vi "Read Environment Options.vi"(8 "error in (no error)":errorcluster, 11 "WebView2 Control in":refnum<class "WebView2 QControl.lvclass">) -> (0 "error out":errorcluster, 2 "Env Options":T1, 3 "WebView2 Control out":refnum<class "WebView2 QControl.lvclass">)   [LabVIEW 2020, in "WebView2 QControl.lvlib" / "WebView2 QControl.lvclass"]
uses:
  WebView2 QControl.lvclass
  WebView2 QControl.lvclass/WebView2 QControl.ctl
  Webview2 Lib/WebView2 Control Object/WebView2 Control.lvclass
  Webview2 Lib/WebView2 Control Object/Core Env Options.ctl
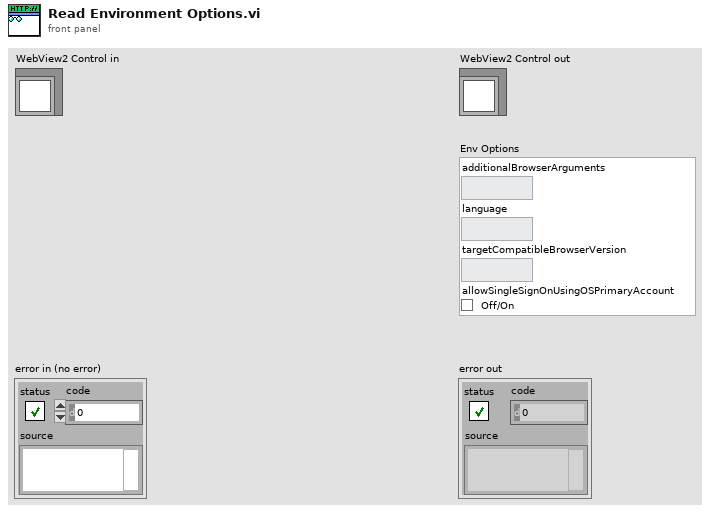
[diagram p1: front panel]
types:
  T1 = typedef "WebView2.lvlib/WebView2 Control.lvclass/Core Env Options.ctl" = cluster{"additionalBrowserArguments":string, "language":string, "targetCompatibleBrowserVersion":string, "allowSingleSignOnUsingOSPrimaryAccount":bool}
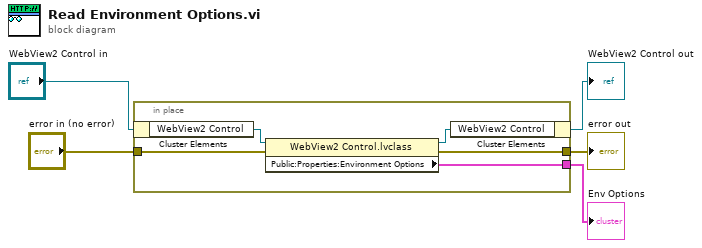
[diagram p0: block diagram]
diagram:
  n1 = in-place {
    in-place-border: "error in (no error)" -> [w10]
    in-place-border: [w9] -> w2
    in-place-border: [w6] -> w1
    n2 = in-place-cluster #1("WebView2 Control in") -> ("WebView2 Control"=w8:refnum<class "WebView2 Control.lvclass">)
    n3 = property class="WebView2 Control.lvclass"(reference=w8, error in=w10) -> (reference out=w7:refnum<class "WebView2 Control.lvclass">, error out=w9:errorcluster, "Public:Properties:Environment Options"=w6:T1)
    n4 = in-place-cluster #1("WebView2 Control"=w7) -> (→"WebView2 Control out":refnum<class "WebView2 QControl.lvclass">)
  }
  "error out" <- w2
  "Env Options" <- w1
